vi "Temperature Reading.vi"() -> ()   [LabVIEW 2020]
panel:
  out "Numeric 2":dbl
  in  "Numeric":dbl
  in  "STOP":bool
  out "Waveform Chart":dbl(graph)
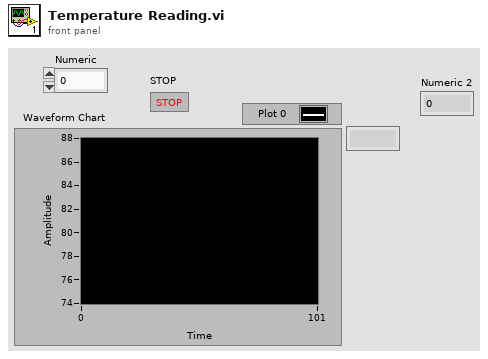
[diagram p1: front panel]
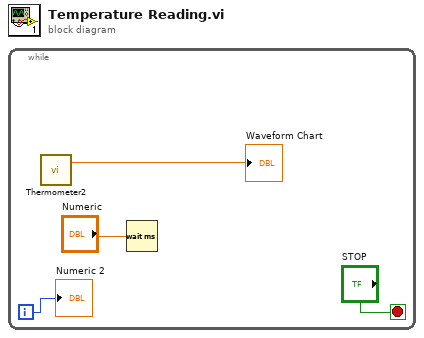
[diagram p0: block diagram]
diagram:
  n1 = while {
    i -> [w1]
    stop <- "STOP" stop-if-true
    n2 = call "Thermometer2.vi"() -> ("Temperature (deg F)"=→"Waveform Chart":dbl)  [unwired: 1 in, 1 out]
    n3 = Wait (ms)(milliseconds to wait="Numeric") -> ()  [unwired: 1 out]
    "Numeric 2" <- w1
  }
